vi "Register New I32 Item.vi"(8 "error in (no error)":errorcluster, 9 "element data type":i32, 10 "Tag Name":string, 11 "Current Value Table in":refnum<class "Current Value Table.lvclass">) -> (0 "error out":errorcluster, 3 "Current Value Table out":refnum<class "Current Value Table.lvclass">)   [LabVIEW 2024, in "Current Value Table.lvlib" / "Current Value Table.lvclass"]
uses:
  Current Value Table.lvclass
  CVT_I32/CVT_I32.lvclass
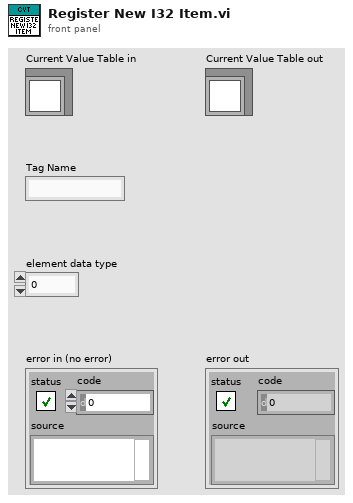
[diagram p1: front panel]
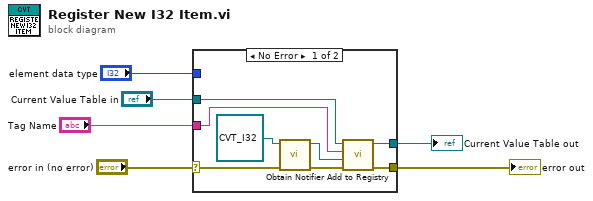
[diagram p0: block diagram]
diagram:
  n1 = case shown="No Error" "error in (no error)" {
    selector: "error in (no error)" -> [w12 w16]
    tunnel: [w10 w16] -> w5
    tunnel: [w8 w15] -> w3
    tunnel: "Current Value Table in" -> [w9 w15]
    tunnel: "element data type" -> [_ _]
    tunnel: "Tag Name" -> [w7 _]
    frame No Error {
      n2 = call-dynamic "Obtain Notifier.vi"("error in (no error)"=w12, "CVT_I32 in"=refnum<class "CVT_I32.lvclass"> refnum) -> ("error out"=w11:errorcluster, "CVT_I32 out"=w14:refnum<class "CVT_I32.lvclass">)  [unwired: 8 in]
      n3 = call-dynamic "Add to Registry.vi"("error in (no error)"=w11, "iCVT_Item in"=w14, "Tag Name"=w7, "Current Value Table in"=w9) -> ("error out"=w10:errorcluster, "Current Value Table out"=w8:refnum<class "Current Value Table.lvclass">)  [unwired: 5 in, 1 out]
    }
    frame Error {
    }
  }
  "error out" <- w5
  "Current Value Table out" <- w3
